vi "Begin.vi"(8 "error in":errorcluster) -> (0 "error out":errorcluster)   [LabVIEW 2018]
doc: "Called before other user functions, this VI is expected to open initial I/O refnums, load in file data, and do all program initialization. Notice that the <B>error out</B> terminal is simply used for data flow. Wiring it to other structures or subVIs ensures that this VI runs first."
uses:
  <vilib>/Rock Robotics/WPI/ThirdParty/Phoenix-LabVIEW/Motor Controller/Controls/CTRE_Phoenix_MotorControl_EnhancedMotorControllerConfigurables.ctl
  <vilib>/Rock Robotics/WPI/ThirdParty/Phoenix-LabVIEW/Motor Controller/Controls/CTRE_Phoenix_MotorControl_BaseConfigurables.ctl
  <vilib>/Rock Robotics/WPI/ThirdParty/Phoenix-LabVIEW/Motor Controller/Controls/CTRE_Phoenix_MotorControl_VelocityMeasurementPeriod.ctl
  <vilib>/Rock Robotics/WPI/ThirdParty/Phoenix-LabVIEW/Motor Controller/Controls/CTRE_Phoenix_MotorControl_SlotStructure.ctl
  <vilib>/Rock Robotics/WPI/ThirdParty/Phoenix-LabVIEW/Motor Controller/Controls/CTRE_Phoenix_MotorControl_FilterStruct.ctl
  <vilib>/Rock Robotics/WPI/ThirdParty/Phoenix-LabVIEW/Motor Controller/Controls/CTRE_Phoenix_MotorControl_RemoteSourceType.ctl
  <vilib>/Rock Robotics/WPI/ThirdParty/Phoenix-LabVIEW/Controls/CTRE_Phoenix_CustomParamConfiguration.ctl
  <vilib>/Rock Robotics/WPI/ThirdParty/Phoenix-LabVIEW/Motor Controller/Controls/CTRE_Phoenix_MotorControl_FeedbackDevice.ctl
  <vilib>/Rock Robotics/WPI/ThirdParty/Phoenix-LabVIEW/Motor Controller/Controls/CTRE_Phoenix_MotorControl_SensorTermFeedbackDevice_Enhanced.ctl
  <vilib>/Rock Robotics/WPI/ThirdParty/Phoenix-LabVIEW/Motor Controller/Controls/CTRE_Phoenix_MotorControl_LimitSwitchNormal.ctl
  <vilib>/Rock Robotics/WPI/ThirdParty/Phoenix-LabVIEW/Motor Controller/Controls/CTRE_Phoenix_MotorControl_LimitSwitchSource_Local.ctl
  <vilib>/Rock Robotics/WPI/SafetyOutput/WPI_SafetyOutputConfigMenu.ctl
  <vilib>/Rock Robotics/WPI/DriverStation/WPI_DriverStationRobotMode2.ctl
  <vilib>/Rock Robotics/WPI/Joystick/WPI_JoystickDeviceEnum.ctl
  <vilib>/Rock Robotics/WPI/Solenoid/WPI_SolenoidChannel.ctl
  <vilib>/Rock Robotics/SystemInterfaces/DIO/FPGA_DIOPWMChannel.ctl
  <vilib>/Rock Robotics/SystemInterfaces/DIO/FPGA_DIOChannel.ctl
  <vilib>/Rock Robotics/WPI/Encoder/WPI_EncoderType.ctl
  Robot Global Data.vi
  <vilib>/Rock Robotics/Network Tables/NT Write String Array.vi
  <vilib>/Rock Robotics/WPI/RobotDrive/WPI_RobotDriveOpen4MotorWithExistingMotors.vi
  <vilib>/Rock Robotics/WPI/Solenoid/WPI_SolenoidOpenDouble.vi
  <vilib>/Rock Robotics/WPI/MotorControl/WPI_MotorControlOpen SPARK.vi
  <vilib>/Rock Robotics/WPI/Switch/WPI_SwitchOpenLimit.vi
  <vilib>/Rock Robotics/WPI/Counter/WPI_CounterDigitalInputToDigitalSource.vi
panel:
  in  "Mag Talon Configs":T1={"Base Configurables"={"openLoopRamp"=0.0, "closedLoopRamp"=0.0, "peakOutputForward"=1.0, "peakOutputReverse"=-1.0, "nominalOutputForward"=0.0, "nominalOutputReverse"=0.0, "neutralDeadband"=0.04, "voltageCompSaturation"=0.0, "voltageMeasurementFilter"=32, "velocityMeasurementPeriod"=100, "velocityMeasurementWindow"=64, "forwardSoftLimitThreshold"=0, "reverseSoftLimitThreshold"=0, "forwardSoftLimitEnable"=FALSE, "reverseSoftLimitEnable"=FALSE, "slot0"={"P"=0.0, "I"=0.0, "D"=0.0, "F"=0.0, "integralZone"=0.0, "allowableClosedLoopError"=0, "maxIntegralAccumulator"=0.0, "closedLoopPeakOutput"=1.0, "closedLoopPeriod"=1}, "slot1"={"P"=0.0, "I"=0.0, "D"=0.0, "F"=0.0, "integralZone"=0.0, "allowableClosedLoopError"=0, "maxIntegralAccumulator"=0.0, "closedLoopPeakOutput"=1.0, "closedLoopPeriod"=1}, "slot2"={"P"=0.0, "I"=0.0, "D"=0.0, "F"=0.0, "integralZone"=0.0, "allowableClosedLoopError"=0, "maxIntegralAccumulator"=0.0, "closedLoopPeakOutput"=1.0, "closedLoopPeriod"=1}, "slot3"={"P"=0.0, "I"=0.0, "D"=0.0, "F"=0.0, "integralZone"=0.0, "allowableClosedLoopError"=0, "maxIntegralAccumulator"=0.0, "closedLoopPeakOutput"=1.0, "closedLoopPeriod"=1}, "auxPIDPolarity"=FALSE, "remoteFilter0"={"remoteSensorDeviceID"=0, "remoteSensorSource"=enum."Off"}, "remoteFilter1"={"remoteSensorDeviceID"=0, "remoteSensorSource"=enum."Off"}, "motionCruiseVelocity"=0, "motionAcceleration"=0, "motionProfileTrajectoryPeriod"=0, "feedbackNotContinuous"=FALSE, "remoteSensorClosedLoopDisableNeutralOnLOS"=FALSE, "clearPositionOnLimitF"=FALSE, "clearPositionOnLimitR"=FALSE, "clearPositionOnQuadIdx"=FALSE, "limitSwitchDisableNeutralOnLOS"=FALSE, "softLimitDisableNeutralOnLOS"=FALSE, "pulseWidthPeriod_EdgesPerRot"=1, "pulseWidthPeriod_FilterWindowSz"=1, "customParam"={"customParam0"=0, "customParam1"=0}, "trajectoryInterpolationEnable"=TRUE}, "primaryPID"={"selectedFeedbackCoefficient"=1.0, "selectedFeedbackSensor"=0}, "auxiliaryPID"={"selectedFeedbackCoefficient"=1.0, "selectedFeedbackSensor"=0}, "sum0Term"=0, "sum1Term"=0, "diff0Term"=0, "diff1Term"=0, "forwardLimitSwitchNormal"=enum."Normally Open", "reverseLimitSwitchNormal"=enum."Normally Open", "forwardLimitSwitchDeviceID"=0, "reverseLimitSwitchDeviceID"=0, "forwardLimitSwitchSource"=enum."Feedback Connector", "reverseLimitSwitchSource"=enum."Feedback Connector", "peakCurrentLimit"=1, "peakCurrentDuration"=1, "continuousCurrentLimit"=1} {"diff1Term" items=["QuadEncoder"=0, "Analog"=2, "Tachometer"=4, "Pulse Width Encoded Position"=8, "Remote Source 0"=11, "Remote Source 1"=12, "Software Emulated"=15]; "diff0Term" items=["QuadEncoder"=0, "Analog"=2, "Tachometer"=4, "Pulse Width Encoded Position"=8, "Remote Source 0"=11, "Remote Source 1"=12, "Software Emulated"=15]; "sum1Term" items=["QuadEncoder"=0, "Analog"=2, "Tachometer"=4, "Pulse Width Encoded Position"=8, "Remote Source 0"=11, "Remote Source 1"=12, "Software Emulated"=15]; "sum0Term" items=["QuadEncoder"=0, "Analog"=2, "Tachometer"=4, "Pulse Width Encoded Position"=8, "Remote Source 0"=11, "Remote Source 1"=12, "Software Emulated"=15]; "auxiliaryPID"."selectedFeedbackSensor" items=["QuadEncoder"=0, "Analog"=2, "Tachometer"=4, "Pulse Width Encoded Position"=8, "Sensor Sum (S0 + S1)"=9, "Sensor Difference (D0 - D1)"=10, "Remote Source 0"=11, "Remote Source 1"=12, "Software Emulated"=15]; "primaryPID"."selectedFeedbackSensor" items=["QuadEncoder"=0, "Analog"=2, "Tachometer"=4, "Pulse Width Encoded Position"=8, "Sensor Sum (S0 + S1)"=9, "Sensor Difference (D0 - D1)"=10, "Remote Source 0"=11, "Remote Source 1"=12, "Software Emulated"=15]; "Base Configurables"."velocityMeasurementPeriod" items=["Period_1ms"=1, "Period_2ms"=2, "Period_5ms"=5, "Period_10ms"=10, "Period_20ms"=20, "Period_25ms"=25, "Period_50ms"=50, "Period_100ms"=100]}
  # "Sum and Diff terms are ways to select more than one sensor as a feedback device. \n Sum 0 is the first feedback device to be used for the Sum term.\n Sum 1 is the feedback device to be added to Sum 0 for the Sum term.\n Diff 0 and Diff 1 work in a similar manner."
  # "These are only applicable\nif using a remote limit switch.\n\nLocal limit switches/no limit\nswitches do not use this."
  # "Current is below Continuous threshold AND\n\n(Requested output is weaker** than applied motor\noutput OR is in the opposite direction).\n/\nMotor output is set to requested output."
  # "Current is above Peak* Threshold for Peak Duration.\n/\nReduce motor output (towards neutral)."
  # "Current is below Continuous threshold.\n/\nRamp motor output towards requested output."
  # "Current is above Continuous threshold.\n/\nReduce motor output (towards neutral)."
  # "Current Limiting is NOT enabled\nby default.\nCall this VI to enable."
  # "*If the configured Peak Threshold is less than the Continuous Threshold, the applied Peak Threshold is set equal to the Configured Continuous Threshold in firmware.\n** Both requested output and applied motor output are in the same direction, and requested output is closer to neutral."
  # "False: Primary Output = PID[0] + PID[1]  ---  Auxiliary Output = PID[0] - PID[1]\nTrue:  Primary Output = PID[0] - PID[1] --- Auxiliary Output = PID[0] + PID[1]"
  # "Enable the motion profile executor to perform linear interpolation between profile points.  Defaults to True."
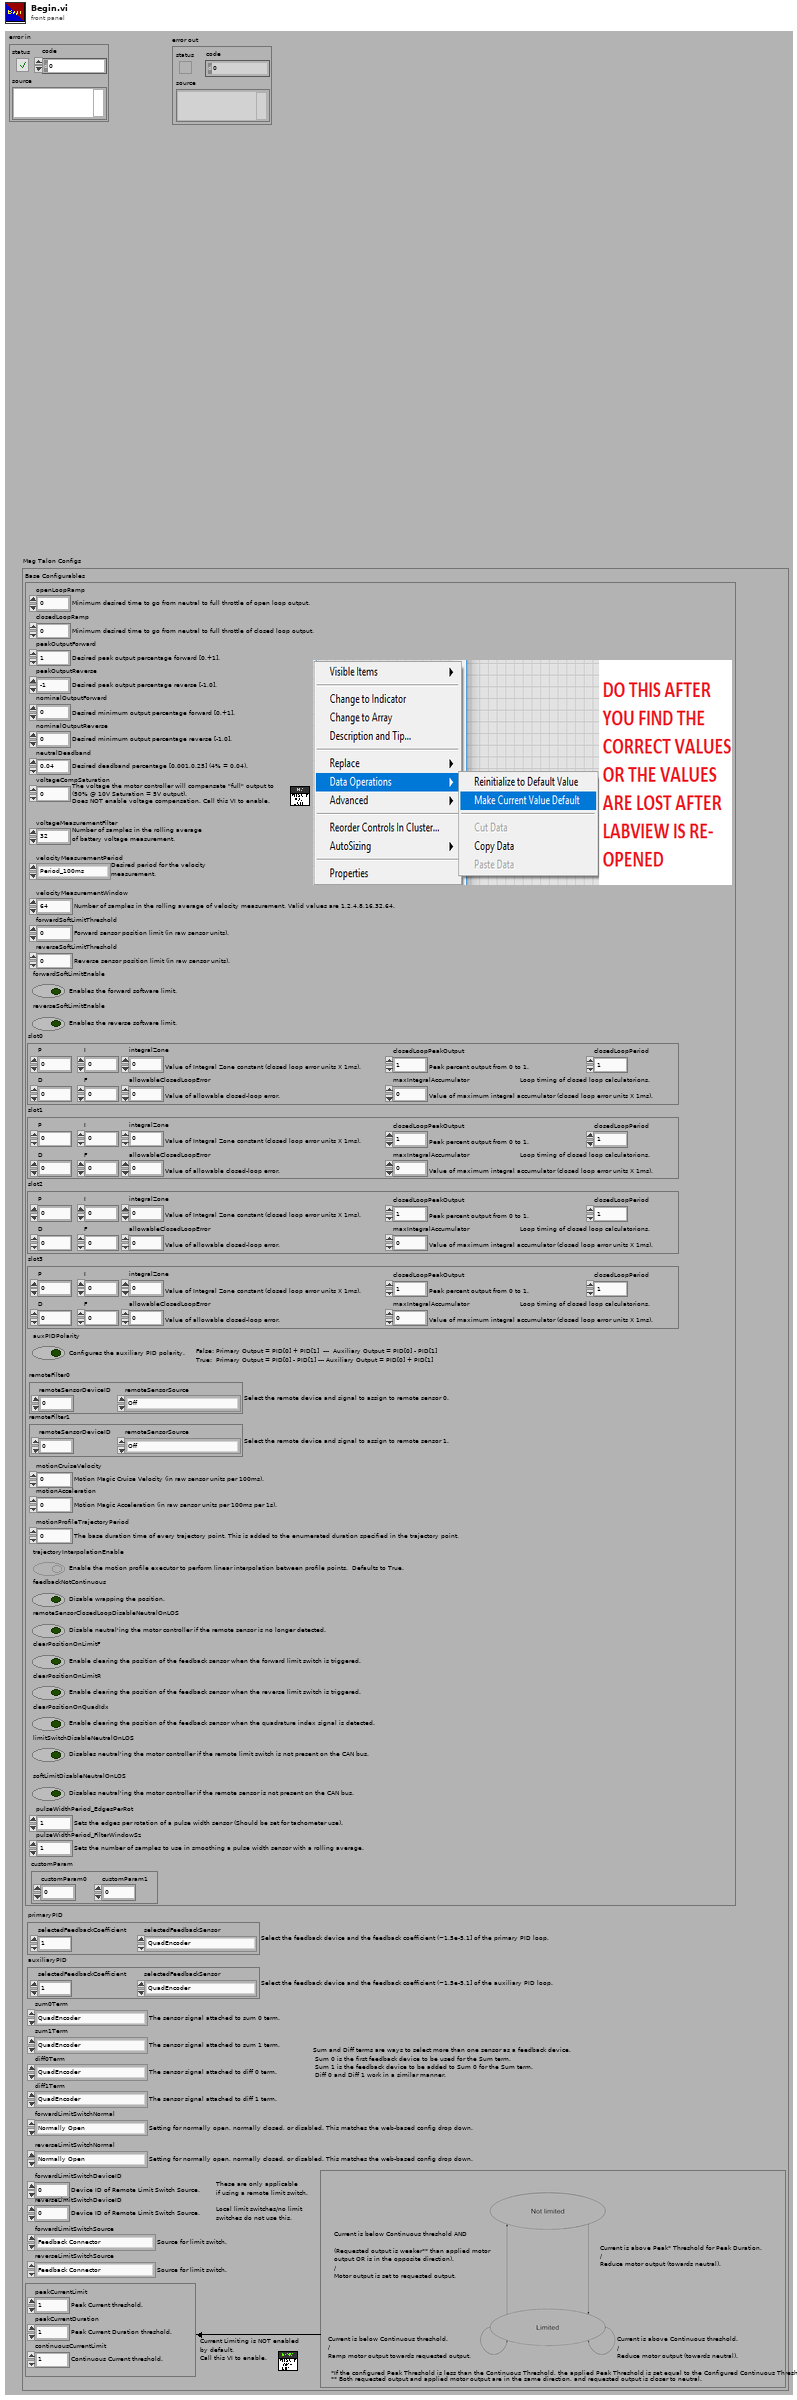
[diagram p1: front panel]
types:
  T1 = typedef "CTRE_Phoenix_MotorControl_EnhancedMotorControllerConfigurables.ctl" = cluster{"Base Configurables":T2, "primaryPID":cluster{"selectedFeedbackCoefficient":dbl, "selectedFeedbackSensor":T8}, "auxiliaryPID":cluster{"selectedFeedbackCoefficient":dbl, "selectedFeedbackSensor":T8}, "sum0Term":T9, "sum1Term":T9, "diff0Term":T9, "diff1Term":T9, "forwardLimitSwitchNormal":T10, "reverseLimitSwitchNormal":T10, "forwardLimitSwitchDeviceID":i32, "reverseLimitSwitchDeviceID":i32, "forwardLimitSwitchSource":T11, "reverseLimitSwitchSource":T11, "peakCurrentLimit":i32, "peakCurrentDuration":i32, "continuousCurrentLimit":i32}
  T2 = typedef "CTRE_Phoenix_MotorControl_BaseConfigurables.ctl" = cluster{"openLoopRamp":dbl, "closedLoopRamp":dbl, "peakOutputForward":dbl, "peakOutputReverse":dbl, "nominalOutputForward":dbl, "nominalOutputReverse":dbl, "neutralDeadband":dbl, "voltageCompSaturation":dbl, "voltageMeasurementFilter":i32, "velocityMeasurementPeriod":T3, "velocityMeasurementWindow":i32, "forwardSoftLimitThreshold":i32, "reverseSoftLimitThreshold":i32, "forwardSoftLimitEnable":bool, "reverseSoftLimitEnable":bool, "slot0":T4, "slot1":T4, "slot2":T4, "slot3":T4, "auxPIDPolarity":bool, "remoteFilter0":T5, "remoteFilter1":T5, "motionCruiseVelocity":i32, "motionAcceleration":i32, "motionProfileTrajectoryPeriod":i32, "feedbackNotContinuous":bool, "remoteSensorClosedLoopDisableNeutralOnLOS":bool, "clearPositionOnLimitF":bool, "clearPositionOnLimitR":bool, "clearPositionOnQuadIdx":bool, "limitSwitchDisableNeutralOnLOS":bool, "softLimitDisableNeutralOnLOS":bool, "pulseWidthPeriod_EdgesPerRot":i32, "pulseWidthPeriod_FilterWindowSz":i32, "customParam":T7, "trajectoryInterpolationEnable":bool}
  T3 = typedef "CTRE_Phoenix_MotorControl_VelocityMeasurementPeriod.ctl" = u16
  T4 = typedef "CTRE_Phoenix_MotorControl_SlotStructure.ctl" = cluster{"P":dbl, "I":dbl, "D":dbl, "F":dbl, "integralZone":dbl, "allowableClosedLoopError":i32, "maxIntegralAccumulator":dbl, "closedLoopPeakOutput":dbl, "closedLoopPeriod":i32}
  T5 = typedef "CTRE_Phoenix_MotorControl_FilterStruct.ctl" = cluster{"remoteSensorDeviceID":u8, "remoteSensorSource":T6}
  T6 = typedef "CTRE_Phoenix_MotorControl_RemoteSourceType.ctl" = enum16{"Off", "Talon SRX Selected Sensor", "Pigeon IMU Yaw", "Pigeon IMU Pitch", "Pigeon IMU Roll", "CANifier Quadrature", "CANifier PWM Input 0", "CANifier PWM Input 1", "CANifier PWM Input 2", "CANifier PWM Input 3", "Gadgeteer Pigeon Yaw", "Gadgeteer Pigeon Pitch", "Gadgeteer Pigeon Roll"}
  T7 = typedef "CTRE_Phoenix_CustomParamConfiguration.ctl" = cluster{"customParam0":i32, "customParam1":i32}
  T8 = typedef "CTRE_Phoenix_MotorControl_FeedbackDevice.ctl" = i8
  T9 = typedef "CTRE_Phoenix_MotorControl_SensorTermFeedbackDevice_Enhanced.ctl" = i8
  T10 = typedef "CTRE_Phoenix_MotorControl_LimitSwitchNormal.ctl" = enum16{"Normally Open", "Normally Closed", "Disabled"}
  T11 = typedef "CTRE_Phoenix_MotorControl_LimitSwitchSource_Local.ctl" = enum16{"Feedback Connector", "Remote Talon SRX", "Remote CANifier", "Deactivated"}
  T12 = typedef "WPI_SolenoidChannel.ctl" = enum8{"Solenoid 0", "Solenoid 1", "Solenoid 2", "Solenoid 3", "Solenoid 4", "Solenoid 5", "Solenoid 6", "Solenoid 7", "Invalid"}
  T13 = typedef "FPGA_DIOPWMChannel.ctl" = enum8{"PWM 0", "PWM 1", "PWM 2", "PWM 3", "PWM 4", "PWM 5", "PWM 6", "PWM 7", "PWM 8", "PWM 9", "PWM MXP 0", "PWM MXP 1", "PWM MXP 2", "PWM MXP 3", "PWM MXP 4", "PWM MXP 5", "PWM MXP 6", "PWM MXP 7", "PWM MXP 8", "PWM MXP 9", "Invalid"}
  T14 = typedef "WPI_EncoderType.ctl" = enum16{"1x", "2x", "4x"}
  T15 = typedef "FPGA_DIOChannel.ctl" = enum8{"DIO 0", "DIO 1", "DIO 2", "DIO 3", "DIO 4", "DIO 5", "DIO 6", "DIO 7", "DIO 8", "DIO 9", "DIO MXP 0", "DIO MXP 1", "DIO MXP 2", "DIO MXP 3", "DIO MXP 4", "DIO MXP 5", "DIO MXP 6", "DIO MXP 7", "DIO MXP 8", "DIO MXP 9", "DIO MXP 10", "DIO MXP 11", "DIO MXP 12", "DIO MXP 13", "DIO MXP 14", "DIO MXP 15", "SPI Port CS1", "SPI Port CS2", "SPI Port CS3", "SPI Port MISO", "SPI Port MOSI", "Invalid"}
  T16 = typedef "WPI_JoystickDeviceEnum.ctl" = enum16{"USB 0", "USB 1", "USB 2", "USB 3", "USB 4", "USB 5"}
  T17 = typedef "WPI_DriverStationRobotMode2.ctl" = enum16{"Autonomous Disabled", "Autonomous Enabled", "Teleop Disabled", "Teleop Enabled", "Disconnected", "Finish", "Test Disabled", "Test Enabled", "Emergency Stopped"}
  T18 = typedef "WPI_SafetyOutputConfigMenu.ctl" = enum16{"Enable", "Disable"}
  T19 = typedef "WPI_DigitalInputDevRef.ctl" = cluster{"DevStatus":errorcluster, "DIO Channel":T15}
  T20 = typedef "FPGA_CounterEncoderSourceConvertionLVSourceType.ctl" = cluster{"DevStatus":errorcluster, "AnalogTriggerMode?":bool, "DigitalMode":cluster{"DIO Channel":T21}, "AnalogTriggerMode":cluster{"AnalogTriggerIndex":T22, "OutputType":T23}}
  T21 = typedef "FPGA_DIODigitalSourceChannel.ctl" = enum8{"DIO 0", "DIO 1", "DIO 2", "DIO 3", "DIO 4", "DIO 5", "DIO 6", "DIO 7", "DIO 8", "DIO 9", "DIO MXP 0", "DIO MXP 1", "DIO MXP 2", "DIO MXP 3", "DIO MXP 4", "DIO MXP 5", "DIO MXP 6", "DIO MXP 7", "DIO MXP 8", "DIO MXP 9", "DIO MXP 10", "DIO MXP 11", "DIO MXP 12", "DIO MXP 13", "DIO MXP 14", "DIO MXP 15", "SPI Port CS1", "SPI Port CS2", "SPI Port CS3", "SPI Port MISO", "SPI Port MOSI", "Disabled"}
  T22 = typedef "FPGA_AnalogTriggerIndex.ctl" = enum8{"Trig 0", "Trig 1", "Trig 2", "Trig 3", "Trig 4", "Trig 5", "Trig 6", "Trig 7", "Invalid"}
  T23 = typedef "FPGA_AnalogTriggerOutType.ctl" = enum16{"InWindow", "TriggerState", "Rising", "Falling"}
  T24 = typedef "WPI_SwitchDevRef.ctl" = cluster{"DevStatus":errorcluster, "DIO Channel":T15, "CntIndex":T25, "Normally Closed":bool}
  T25 = typedef "FPGA_CounterCtrSystemIndex.ctl" = enum8{"Ctr 0", "Ctr 1", "Ctr 2", "Ctr 3", "Ctr 4", "Ctr 5", "Ctr 6", "Ctr 7", "Invalid"}
  T26 = typedef "WPI_MotorControlDeviceRef.ctl" = cluster{"DeviceStatus":errorcluster, "Type":T27, "PWM":cluster{"PWM Channel":T13, "DeadBand":T28}, "CAN":cluster{"Device Number":u8, "SetOutput VI Ref":variant, "GetOutput VI Ref":variant, "Enable VI Ref":variant, "Disable VI Ref":variant, "Data":variant}, "Invert":bool, "DIO PWM":cluster{"PWM \"Enable\" Channel":T13, "DIOChannel":T15, "PWM Rate":dbl}}
  T27 = typedef "WPI_MotorControlType.ctl" = enum16{"PWM", "CAN", "DIO PWM"}
  T28 = typedef "WPI_PWMDeadband.ctl" = cluster{"Name":string, "maxPositivePwm":i32, "minPositivePwm":i32, "centerPwm":i32, "maxNegativePwm":i32, "minNegativePwm":i32, "angularRange":u16}
  T29 = typedef "WPI_EncoderDevRef.ctl" = cluster{"DevStatus":errorcluster, "EncoderIndex":T30, "CounterIndex":T25, "DistancePerCount":dbl, "Decoding Type":T14}
  T30 = typedef "FPGA_EncoderIdx.ctl" = enum8{"Enc 0", "Enc 1", "Enc 2", "Enc 3", "Enc 4", "Enc 5", "Enc 6", "Enc 7", "Invalid"}
  T31 = typedef "WPI_JoystickDevRef.ctl" = cluster{"Device":T16}
  T32 = typedef "WPI_RobotDriveDevRef.ctl" = cluster{"DevStatus":errorcluster, "Motors[]":T26[], "Square Inputs":bool, "Max Output":dbl}
  T33 = typedef "WPI_ServoDeviceRef.ctl" = cluster{"DeviceStatus":errorcluster, "PWM Channel":T13, "DeadBand":T28}
  T34 = typedef "WPI_SolenoidDevRef.ctl" = cluster{"DevStatus":errorcluster, "Pneumatics Control Module":u8, "Forward Solenoid Channel":T12, "Reverse Solenoid Channel":T12}
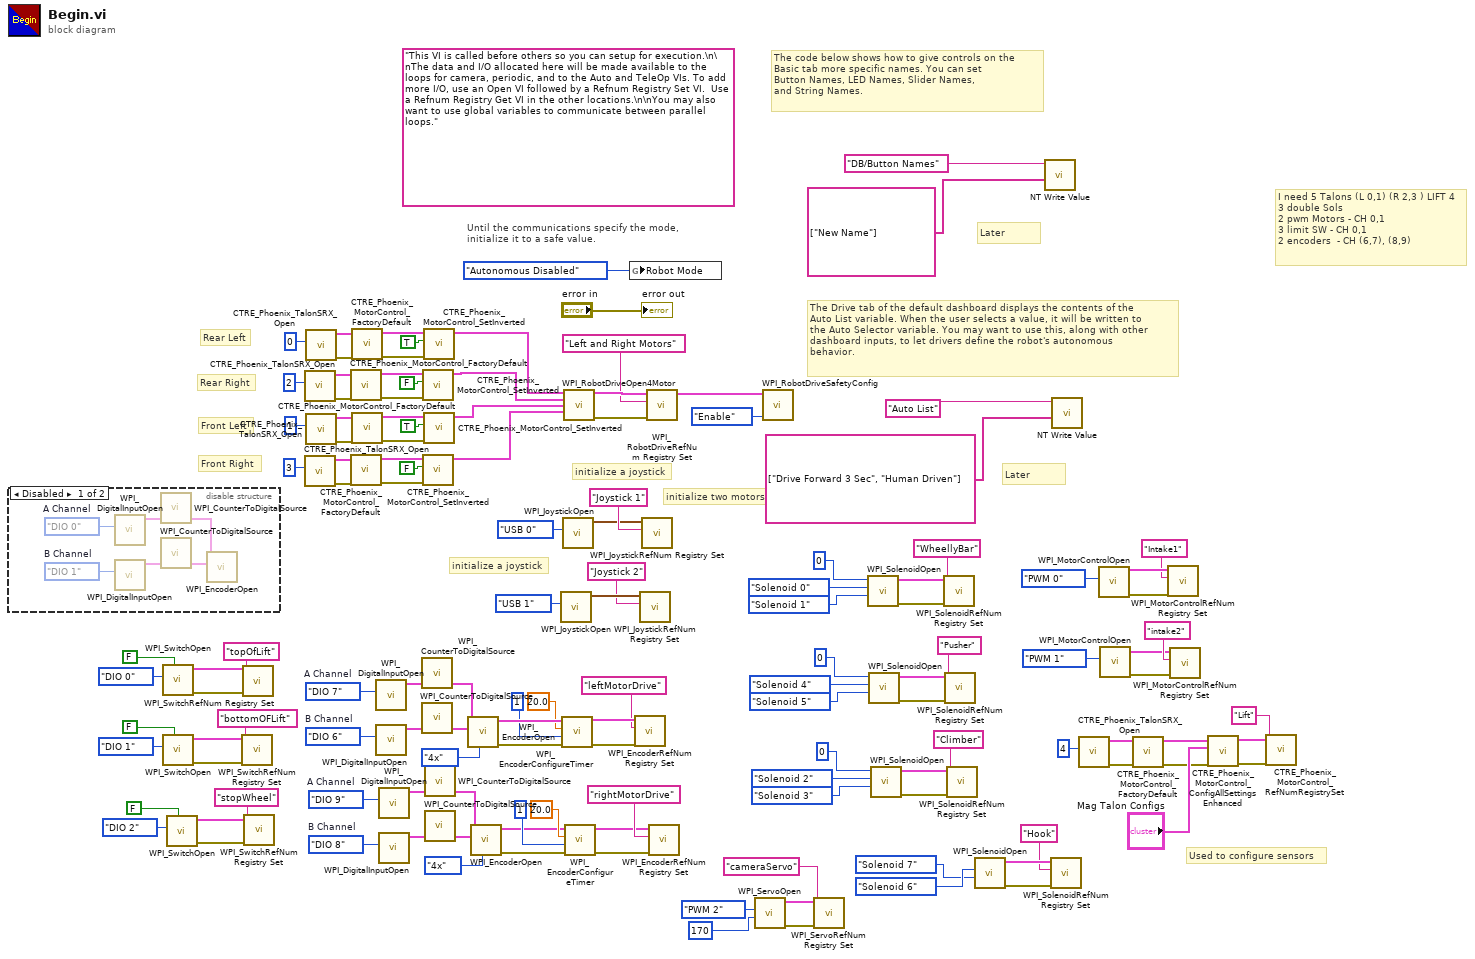
[diagram p0: block diagram]
diagram:
  w24 = FPGA_DIOChannel."DIO 8"  # B Channel
  w25 = FPGA_DIOChannel."DIO 9"  # A Channel
  w45 = FPGA_DIOChannel."DIO 6"  # B Channel
  w44 = FPGA_DIOChannel."DIO 7"  # A Channel
  (unwired) "This VI is called before others so you can setup for execution.\n\nThe data and I/O allocated here will be made available to the loops for camera, periodic, and to the Auto and TeleOp VIs. To add more I/O, use an Open VI followed by a Refnum Registry Set VI.  Use a Refnum Registry Get VI in the other locations.\n\nYou may also want to use global variables to communicate between parallel loops."
  # "Used to configure sensors"
  # "Front Right"
  # "Front Left"
  # "Rear Right"
  # "Rear Left"
  # "Later"
  # "initialize a joystick"
  # "Later"
  # "I need 5 Talons (L 0,1) (R 2,3 ) LIFT 4\n3 double Sols\n2 pwm Motors - CH 0,1\n3 limit SW - CH 0,1 \n2 encoders  - CH (6,7), (8,9)"
  # "The Drive tab of the default dashboard displays the contents of the\nAuto List variable. When the user selects a value, it will be written to\nthe Auto Selector variable. You may want to use this, along with other\ndashboard inputs, to let drivers define the robot's autonomous\nbehavior."
  # "The code below shows how to give controls on the\nBasic tab more specific names. You can set\nButton Names, LED Names, Slider Names,\nand String Names."
  # "initialize a joystick"
  # "Until the communications specify the mode,\ninitialize it to a safe value."
  # "initialize two motors"
  n1 = disable-structure shown="Disabled" {
    frame Disabled {
      w139 = FPGA_DIOChannel."DIO 1"  # B Channel
      w138 = FPGA_DIOChannel."DIO 0"  # A Channel
      n2 = call <vilib>:"WPI_DigitalInputOpen.vi"("DIO Channel"=w138) -> ("DigitalInputDevRef"=w135:T19)  [unwired: 1 in, 9 out]
      n3 = call <vilib>:"WPI_DigitalInputOpen.vi"("DIO Channel"=w139) -> ("DigitalInputDevRef"=w136:T19)  [unwired: 1 in, 9 out]
      n4 = call-poly <vilib>:"WPI_CounterToDigitalSource.vi"("DigitalInputDevRef"=w135) -> ("Digital Source"=w134:T20)  [unwired: 6 out]
      n5 = call-poly <vilib>:"WPI_CounterToDigitalSource.vi"("DigitalInputDevRef"=w136) -> ("Digital Source"=w137:T20)  [unwired: 6 out]
      n6 = call <vilib>:"WPI_EncoderOpen.vi"("BSource"=w137, "ASource"=w134) -> ()  [unwired: 6 in, 4 out]
    }
    frame Enabled {
    }
  }
  n7 = call-poly <vilib>:"WPI_SwitchOpen.vi"("Normally Closed"=FALSE, "DIO Channel"=FPGA_DIOChannel."DIO 0") -> ("error out"=w54:errorcluster, "SwitchDevRef"=w53:T24)  [unwired: 8 in]
  n8 = call-poly <vilib>:"WPI_SwitchOpen.vi"("Normally Closed"=FALSE, "DIO Channel"=FPGA_DIOChannel."DIO 1") -> ("error out"=w51:errorcluster, "SwitchDevRef"=w52:T24)  [unwired: 8 in]
  n9 = call-poly <vilib>:"WPI_SwitchOpen.vi"("Normally Closed"=FALSE, "DIO Channel"=FPGA_DIOChannel."DIO 2") -> ("error out"=w49:errorcluster, "SwitchDevRef"=w50:T24)  [unwired: 8 in]
  n10 = call <vilib>:"WPI_SwitchRefNum Registry Set.vi"("error in (no error)"=w51, "refnum name"="bottomOFLift", "SwitchDevRef"=w52) -> ()  [unwired: 7 in, 2 out]
  n11 = call <vilib>:"WPI_SwitchRefNum Registry Set.vi"("error in (no error)"=w54, "refnum name"="topOfLift", "SwitchDevRef"=w53) -> ()  [unwired: 7 in, 2 out]
  n12 = call <vilib>:"WPI_SwitchRefNum Registry Set.vi"("error in (no error)"=w49, "refnum name"="stopWheel", "SwitchDevRef"=w50) -> ()  [unwired: 7 in, 2 out]
  n13 = call <vilib>:"CTRE_Phoenix_TalonSRX_Open.vi"("Device Number"=u8 2) -> ("error out"=w105:errorcluster, "CAN Talon SRX Ref"=w106:T26)  [unwired: 9 in]
  n14 = call <vilib>:"CTRE_Phoenix_TalonSRX_Open.vi"("Device Number"=u8 3) -> ("error out"=w93:errorcluster, "CAN Talon SRX Ref"=w94:T26)  [unwired: 9 in]
  n15 = call <vilib>:"CTRE_Phoenix_TalonSRX_Open.vi"("Device Number"=u8 0) -> ("error out"=w116:errorcluster, "CAN Talon SRX Ref"=w115:T26)  [unwired: 9 in]
  n16 = call <vilib>:"CTRE_Phoenix_TalonSRX_Open.vi"("Device Number"=u8 1) -> ("error out"=w104:errorcluster, "CAN Talon SRX Ref"=w103:T26)  [unwired: 9 in]
  n17 = call <vilib>:"CTRE_Phoenix_MotorControl_FactoryDefault.vi"("error in"=w105, "PhoenixMotorControlDevRef"=w106) -> ("error out"=w107:errorcluster, "PhoenixMotorControlDevRef"=w108:T26)  [unwired: 8 in]
  n18 = call <vilib>:"CTRE_Phoenix_MotorControl_FactoryDefault.vi"("error in"=w93, "PhoenixMotorControlDevRef"=w94) -> ("error out"=w95:errorcluster, "PhoenixMotorControlDevRef"=w96:T26)  [unwired: 8 in]
  n19 = call <vilib>:"CTRE_Phoenix_MotorControl_FactoryDefault.vi"("error in"=w116, "PhoenixMotorControlDevRef"=w115) -> ("error out"=w114:errorcluster, "PhoenixMotorControlDevRef"=w113:T26)  [unwired: 8 in]
  n20 = call <vilib>:"CTRE_Phoenix_MotorControl_FactoryDefault.vi"("error in"=w104, "PhoenixMotorControlDevRef"=w103) -> ("error out"=w102:errorcluster, "PhoenixMotorControlDevRef"=w101:T26)  [unwired: 8 in]
  n21 = call <vilib>:"WPI_DigitalInputOpen.vi"("DIO Channel"=w44) -> ("DigitalInputDevRef"=w41:T19)  [unwired: 1 in, 9 out]
  n22 = call <vilib>:"WPI_DigitalInputOpen.vi"("DIO Channel"=w45) -> ("DigitalInputDevRef"=w42:T19)  [unwired: 1 in, 9 out]
  n23 = call <vilib>:"WPI_DigitalInputOpen.vi"("DIO Channel"=w25) -> ("DigitalInputDevRef"=w28:T19)  [unwired: 1 in, 9 out]
  n24 = call <vilib>:"WPI_DigitalInputOpen.vi"("DIO Channel"=w24) -> ("DigitalInputDevRef"=w27:T19)  [unwired: 1 in, 9 out]
  n25 = call-poly <vilib>:"WPI_CounterToDigitalSource.vi"("DigitalInputDevRef"=w41) -> ("Digital Source"=w40:T20)  [unwired: 6 out]
  n26 = call-poly <vilib>:"WPI_CounterToDigitalSource.vi"("DigitalInputDevRef"=w42) -> ("Digital Source"=w43:T20)  [unwired: 6 out]
  n27 = call <vilib>:"CTRE_Phoenix_MotorControl_SetInverted.vi"("error in (no error)"=w107, "Invert?"=FALSE, "PhoenixMotorControlDevRef"=w108) -> ("PhoenixMotorControlDevRef"=w91:T26)  [unwired: 7 in, 1 out]
  n28 = call <vilib>:"CTRE_Phoenix_MotorControl_SetInverted.vi"("error in (no error)"=w95, "Invert?"=FALSE, "PhoenixMotorControlDevRef"=w96) -> ("PhoenixMotorControlDevRef"=w89:T26)  [unwired: 7 in, 1 out]
  n29 = call <vilib>:"CTRE_Phoenix_MotorControl_SetInverted.vi"("error in (no error)"=w114, "Invert?"=TRUE, "PhoenixMotorControlDevRef"=w113) -> ("PhoenixMotorControlDevRef"=w92:T26)  [unwired: 7 in, 1 out]
  n30 = call <vilib>:"CTRE_Phoenix_MotorControl_SetInverted.vi"("error in (no error)"=w102, "Invert?"=TRUE, "PhoenixMotorControlDevRef"=w101) -> ("PhoenixMotorControlDevRef"=w90:T26)  [unwired: 7 in, 1 out]
  n31 = call-poly <vilib>:"WPI_CounterToDigitalSource.vi"("DigitalInputDevRef"=w28) -> ("Digital Source"=w29:T20)  [unwired: 6 out]
  n32 = call-poly <vilib>:"WPI_CounterToDigitalSource.vi"("DigitalInputDevRef"=w27) -> ("Digital Source"=w26:T20)  [unwired: 6 out]
  n33 = call <vilib>:"WPI_EncoderOpen.vi"("Decoding Type"=WPI_EncoderType."4x", "BSource"=w43, "ASource"=w40) -> ("error out"=w38:errorcluster, "EncoderDevRef"=w39:T29)  [unwired: 5 in, 2 out]
  n34 = call <vilib>:"WPI_EncoderOpen.vi"("Decoding Type"=WPI_EncoderType."4x", "BSource"=w26, "ASource"=w29) -> ("error out"=w31:errorcluster, "EncoderDevRef"=w30:T29)  [unwired: 5 in, 2 out]
  n35 = call <vilib>:"WPI_JoystickOpen.vi"("JoystickDevice"=WPI_JoystickDeviceEnum."USB 1") -> ("JoystickDevRef"=w118:T31)  [unwired: 10 in]
  n36 = call <vilib>:"WPI_EncoderConfigureTimer.vi"("error in (no error)"=w38, "Number Samples to Average"=u8 1, "Minimum Rate"=20.0, "EncoderDevRef"=w39) -> ("error out"=w22:errorcluster, "EncoderDevRef"=w23:T29)  [unwired: 6 in]
  n37 = call <vilib>:"WPI_JoystickOpen.vi"("JoystickDevice"=WPI_JoystickDeviceEnum."USB 0") -> ("JoystickDevRef"=w126:T31)  [unwired: 10 in]
  n38 = call-poly <vilib>:"WPI_RobotDriveOpen4Motor.vi"("Rear Left Motor Dev Ref"=w92, "Rear Right Motor Dev Ref"=w91, "Front Left Motor Dev Ref"=w90, "Front Right Motor Dev Ref"=w89) -> ("RobotDriveDevRef"=w133:T32, "error out"=w131:errorcluster)  [unwired: 10 in]
  n39 = call <vilib>:"WPI_EncoderConfigureTimer.vi"("error in (no error)"=w31, "Number Samples to Average"=u8 1, "Minimum Rate"=20.0, "EncoderDevRef"=w30) -> ("error out"=w18:errorcluster, "EncoderDevRef"=w19:T29)  [unwired: 6 in]
  n40 = global write "Robot Global Data.vi" "Robot Mode"(WPI_DriverStationRobotMode2."Autonomous Disabled" ("Robot Mode")) -> ()
  n41 = call <vilib>:"WPI_EncoderRefNum Registry Set.vi"("error in (no error)"=w22, "refnum name"="leftMotorDrive", "EncoderDevRef"=w23) -> ()  [unwired: 7 in, 2 out]
  n42 = call <vilib>:"WPI_JoystickRefNum Registry Set.vi"("refnum name"="Joystick 2", "JoystickDevRef"=w118) -> ()  [unwired: 8 in, 2 out]
  n43 = call <vilib>:"WPI_JoystickRefNum Registry Set.vi"("refnum name"="Joystick 1", "JoystickDevRef"=w126) -> ()  [unwired: 8 in, 2 out]
  n44 = call <vilib>:"WPI_RobotDriveRefNum Registry Set.vi"("error in (no error)"=w131, "refnum name"="Left and Right Motors", "RobotDriveDevRef"=w133) -> ("RobotDriveDevRef"=w130:T32)  [unwired: 1 in, 7 out]
  n45 = call <vilib>:"WPI_EncoderRefNum Registry Set.vi"("error in (no error)"=w18, "refnum name"="rightMotorDrive", "EncoderDevRef"=w19) -> ()  [unwired: 7 in, 2 out]
  n46 = call <vilib>:"WPI_ServoOpen.vi"("Angular Range"=u16 170, "PWM Channel"=FPGA_DIOPWMChannel."PWM 2") -> ("error out"=w14:errorcluster, "ServoDeviceRef"=w15:T33)  [unwired: 8 in]
  n47 = call <vilib>:"WPI_RobotDriveSafetyConfig.vi"("mode"=WPI_SafetyOutputConfigMenu."Enable", "RobotDriveDevRef"=w130) -> ()  [unwired: 8 in, 2 out]
  n48 = call <vilib>:"WPI_ServoRefNum Registry Set.vi"("error in (no error)"=w14, "refnum name"="cameraServo", "ServoDeviceRef"=w15) -> ()  [unwired: 7 in, 2 out]
  n49 = call-poly <vilib>:"WPI_SolenoidOpen.vi"("Reverse Solenoid Channel"=WPI_SolenoidChannel."Solenoid 1", "Forward Solenoid Channel"=WPI_SolenoidChannel."Solenoid 0", "Pneumatics Control Module (0)"=u8 0) -> ("error out"=w84:errorcluster, "SolenoidDevRef"=w85:T34)  [unwired: 7 in]
  n50 = call-poly <vilib>:"WPI_SolenoidOpen.vi"("Reverse Solenoid Channel"=WPI_SolenoidChannel."Solenoid 5", "Forward Solenoid Channel"=WPI_SolenoidChannel."Solenoid 4", "Pneumatics Control Module (0)"=u8 0) -> ("error out"=w81:errorcluster, "SolenoidDevRef"=w80:T34)  [unwired: 7 in]
  n51 = call-poly <vilib>:"WPI_SolenoidOpen.vi"("Reverse Solenoid Channel"=WPI_SolenoidChannel."Solenoid 3", "Forward Solenoid Channel"=WPI_SolenoidChannel."Solenoid 2", "Pneumatics Control Module (0)"=u8 0) -> ("error out"=w72:errorcluster, "SolenoidDevRef"=w73:T34)  [unwired: 7 in]
  n52 = call <vilib>:"WPI_SolenoidRefNum Registry Set.vi"("error in (no error)"=w84, "refnum name"="WheellyBar", "SolenoidDevRef"=w85) -> ()  [unwired: 7 in, 2 out]
  n53 = call <vilib>:"WPI_SolenoidRefNum Registry Set.vi"("error in (no error)"=w81, "refnum name"="Pusher", "SolenoidDevRef"=w80) -> ()  [unwired: 7 in, 2 out]
  n54 = call <vilib>:"WPI_SolenoidRefNum Registry Set.vi"("error in (no error)"=w72, "refnum name"="Climber", "SolenoidDevRef"=w73) -> ()  [unwired: 7 in, 2 out]
  n55 = call-poly <vilib>:"WPI_SolenoidOpen.vi"("Reverse Solenoid Channel"=WPI_SolenoidChannel."Solenoid 7", "Forward Solenoid Channel"=WPI_SolenoidChannel."Solenoid 6" ("Reverse Solenoid Channel")) -> ("error out"=w5:errorcluster, "SolenoidDevRef"=w4:T34)  [unwired: 8 in]
  n56 = call-poly <vilib>:"NT Write Value.vi"("String Array"=string[] ["New Name"], "Name"="DB/Button Names") -> ()  [unwired: 9 in, 1 out]
  n57 = call <vilib>:"WPI_SolenoidRefNum Registry Set.vi"("error in (no error)"=w5, "refnum name"="Hook", "SolenoidDevRef"=w4) -> ()  [unwired: 7 in, 2 out]
  n58 = call-poly <vilib>:"NT Write Value.vi"("String Array"=string[] ["Drive Forward 3 Sec", "Human Driven"], "Name"="Auto List") -> ()  [unwired: 9 in, 1 out]
  n59 = call <vilib>:"CTRE_Phoenix_TalonSRX_Open.vi"("Device Number"=u8 4) -> ("error out"=w10:errorcluster, "CAN Talon SRX Ref"=w11:T26)  [unwired: 9 in]
  n60 = call-poly <vilib>:"WPI_MotorControlOpen.vi"("PWM Channel"=FPGA_DIOPWMChannel."PWM 0") -> ("error out"=w67:errorcluster, "MotorControlDeviceRef"=w68:T26)  [unwired: 9 in]
  n61 = call-poly <vilib>:"WPI_MotorControlOpen.vi"("PWM Channel"=FPGA_DIOPWMChannel."PWM 1") -> ("error out"=w63:errorcluster, "MotorControlDeviceRef"=w64:T26)  [unwired: 9 in]
  n62 = call <vilib>:"CTRE_Phoenix_MotorControl_FactoryDefault.vi"("error in"=w10, "PhoenixMotorControlDevRef"=w11) -> ("error out"=w8:errorcluster, "PhoenixMotorControlDevRef"=w9:T26)  [unwired: 8 in]
  n63 = call <vilib>:"WPI_MotorControlRefNum Registry Set.vi"("error in (no error)"=w67, "refnum name"="Intake1", "MotorControlDevRef"=w68) -> ()  [unwired: 7 in, 2 out]
  n64 = call <vilib>:"WPI_MotorControlRefNum Registry Set.vi"("error in (no error)"=w63, "refnum name"="intake2", "MotorControlDevRef"=w64) -> ()  [unwired: 7 in, 2 out]
  n65 = call <vilib>:"CTRE_Phoenix_MotorControl_ConfigAllSettingsEnhanced.vi"("error in (no error)"=w8, "Enhanced Motor Controller Configurables"="Mag Talon Configs", "PhoenixMotorControlDevRef"=w9) -> ("error out"=w6:errorcluster, "PhoenixMotorControlDevRef"=w7:T26)  [unwired: 7 in]
  n66 = call <vilib>:"CTRE_Phoenix_MotorControl_RefNumRegistrySet.vi"("error in (no error)"=w6, "refnum name"="Lift", "PhoenixMotorControlDevRef"=w7) -> ()  [unwired: 7 in, 2 out]
  "error out" <- "error in"
